vi "draw.vi"(0 "reference":refnum<class "StateNode.lvclass">, 1 "graphics":refnum<class "Graphics.lvclass">, 5 "error in (no error)":errorcluster) -> (14 "reference out":refnum<class "StateNode.lvclass">, 19 "error out":errorcluster)   [LabVIEW 2014, in "StateNode.lvclass"]
doc: "public void draw(Graphics2D g2, Point2D p, Point2D q)"
uses:
  <resource>/Framework/Providers/Open_GDS/UML/StateNode_class/StateNode.lvclass
  <resource>/Framework/Providers/Open_GDS/UML/Graphics_class/Graphics.lvclass
  <resource>/Framework/Providers/Open_GDS/UML/General/Point/Point Point2D.ctl
  <resource>/Framework/Providers/Open_GDS/UML/UMLEditor/UMLEditor_StoredColors.ctl
  <resource>/Framework/Providers/Open_GDS/UML/MultiLineString_class/MultiLineString.lvclass
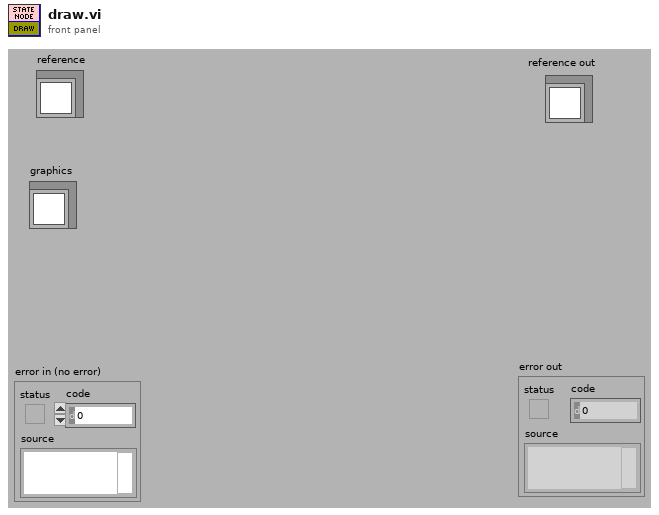
[diagram p1: front panel]
types:
  T1 = typedef "UMLEditor_StoredColors.ctl" = enum16{"ClassBackgroudColor", "ClassBackgroudColorWithClassPath", "ClassBackgroudColorForApplicationVIStereotype", "ClassBackgroudColorForTypeStereotype", "StateBackgroudColor"}
  T2 = typedef "Point Point2D.ctl" = cluster{"x":dbl, "y":dbl}
  T3 = typedef "StateNode.lvclass/ObjectAttributes.ctl" = cluster{"Base class":T4, "state":refnum<class "MultiLineString.lvclass">, "action":refnum<class "MultiLineString.lvclass">, "DEFAULT_WIDTH":i32, "DEFAULT_HEIGHT":i32}
  T4 = typedef "RectangularNode.lvclass/ObjectAttributes.ctl" = cluster{"Base class":T5, "bounds":T6}
  T5 = typedef "AbstractNode.lvclass/ObjectAttributes.ctl" = cluster{"parent":refnum<class "AbstractNode.lvclass">, "children":refnum<class "AbstractNode.lvclass">[], "Hidden":bool}
  T6 = typedef "Rectangle Rectangle2D.ctl" = cluster{"x":dbl, "y":dbl, "width":dbl, "height":dbl}
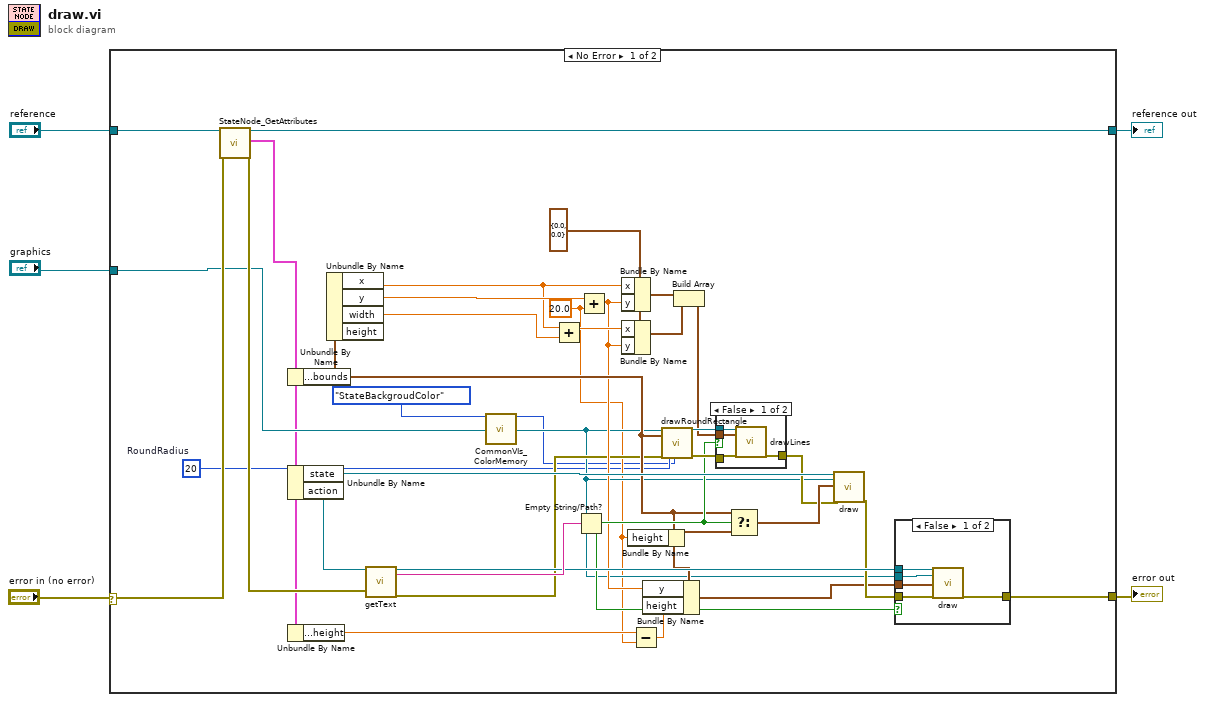
[diagram p0: block diagram]
diagram:
  n1 = case shown="No Error" "error in (no error)" {
    selector: "error in (no error)" -> [w16 w53]
    tunnel: "reference" -> [w41 w54]
    tunnel: [w15 w53] -> w4
    tunnel: [w40 w54] -> w3
    tunnel: "graphics" -> [w13 _]
    frame No Error {
      w8 = i16 20  # RoundRadius
      w27 = T2 {"x"=0.0, "y"=0.0} ("point2D")
      w9 = 20.0 ("y")
      n2 = call <resource>:"StateNode_GetAttributes.vi"("reference in"=w41, "error in (no error)"=w16) -> ("reference out"=w40:refnum<class "StateNode.lvclass">, "Attributes"=w12:T3, "error out"=w38:errorcluster)  [unwired: 15 out]
      n3 = Unbundle By Name(w12) -> ("Base class.bounds"=w19:T6)
      n4 = Unbundle By Name(w12) -> ("state"=w39:refnum<class "MultiLineString.lvclass">, "action"=w37:refnum<class "MultiLineString.lvclass">)
      n5 = Unbundle By Name(w12) -> ("Base class.bounds.height"=w11:dbl)
      n6 = Unbundle By Name(w19) -> ("x"=w26:dbl, "y"=w28:dbl, "width"=w25:dbl)  [unwired: 1 out]
      n7 = call-dynamic "getText.vi"("reference"=w37, "error in (no error)"=w38) -> ("reference out"=w34:refnum<class "MultiLineString.lvclass">, "text"=w36:string, "error out"=w17:errorcluster)  [unwired: 15 in]
      n8 = call <resource>:"CommonVIs_ColorMemory.vi"("ColorName"=UMLEditor_StoredColors."StateBackgroudColor" ("UMLPathes")) -> ("Color Out"=w6:u32)  [unwired: 3 in, 15 out]
      n9 = Add(x=w26, y=w25) -> (x+y=w24:dbl)
      n10 = Empty String/Path?(string/path=w36) -> (empty?=w30:bool)
      n11 = Add(x=w28, y=w9) -> (x+y=w18:dbl)
      n12 = Bundle By Name(cluster=w27, "x"=w26, "y"=w18) -> (w23:T2)
      n13 = Bundle By Name(cluster=w27, "x"=w24, "y"=w18) -> (w22:T2)
      n14 = Bundle By Name(cluster=w19, "height"=w9) -> (w20:T6)
      n15 = Subtract(x=w11, y=w9) -> (x-y=w10:dbl)
      n16 = Bundle By Name(cluster=w19, "y"=w18, "height"=w10) -> (w14:T6)
      n17 = call-dynamic "drawRoundRectangle.vi"("reference"=w13, "rectangle"=w19, "error in (no error)"=w17, "RoundRadius"=w8, "FillClor(if not used=BorderColorIsUsed,AutoFill)"=w6) -> ("reference out"=w32:refnum<class "Graphics.lvclass">, "error out"=w31:errorcluster)  [unwired: 13 in]
      n18 = Build Array(w23, w22) -> (w21:T2[])
      n19 = case shown="False" w30 {
        tunnel: w32 -> [w45 _]
        tunnel: w31 -> [w44 w46]
        tunnel: [w43 w46] -> w29
        tunnel: w21 -> [w42 _]
        frame False {
          n20 = call <resource>:"drawLines.vi"("reference"=w45, "points"=w42, "error in (no error)"=w44) -> ("error out"=w43:errorcluster)  [unwired: 4 in, 12 out]
        }
        frame True {
        }
      }
      n21 = Select(t=w19, s=w30, f=w20) -> (s? t:f=w35:T6)
      n22 = call-dynamic "draw.vi"("reference"=w39, "graphics"=w13, "bounds"=w35, "error in (no error)"=w29) -> ("error out"=w33:errorcluster)  [unwired: 14 in, 1 out]
      n23 = case shown="False" w30 {
        tunnel: w34 -> [w51 _]
        tunnel: w13 -> [w50 _]
        tunnel: w33 -> [w49 w52]
        tunnel: [w48 w52] -> w15
        tunnel: w14 -> [w47 _]
        frame False {
          n24 = call-dynamic "draw.vi"("reference"=w51, "graphics"=w50, "bounds"=w47, "error in (no error)"=w49) -> ("error out"=w48:errorcluster)  [unwired: 14 in, 1 out]
        }
        frame True {
        }
      }
    }
    frame Error {
    }
  }
  "reference out" <- w3
  "error out" <- w4
